vi "LE 4 Byte Array to fp32 (Subvi).vi"(9 "4 Bytes in":u8[](array[numeric])) -> (3 "fp32 Out":sgl)   [LabVIEW 2019]
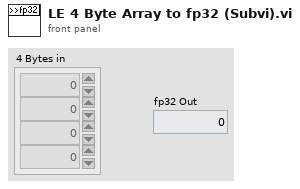
[diagram p1: front panel]
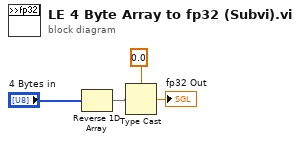
[diagram p0: block diagram]
diagram:
  n1 = Reverse 1D Array(array="4 Bytes in") -> (reversed array=w4:u8[])
  n2 = Type Cast(type=sgl 0.0, x=w4) -> (*(type *) &x=→"fp32 Out":sgl)
